vi "Read VISA address.vi"(8 "error in (no error)":errorcluster, 11 "PS Driver in":refnum<class "PS Driver.lvclass">) -> (0 "error out":errorcluster, 2 "VISA address":refnum<visa-resource-name>="GPIB0::22::INSTR", 3 "PS Driver out":refnum<class "PS Driver.lvclass">)   [LabVIEW 2021, in "PS Driver.lvlib" / "PS Driver.lvclass"]
uses:
  PS Driver.lvclass
  PS Driver.lvclass/PS Driver.ctl
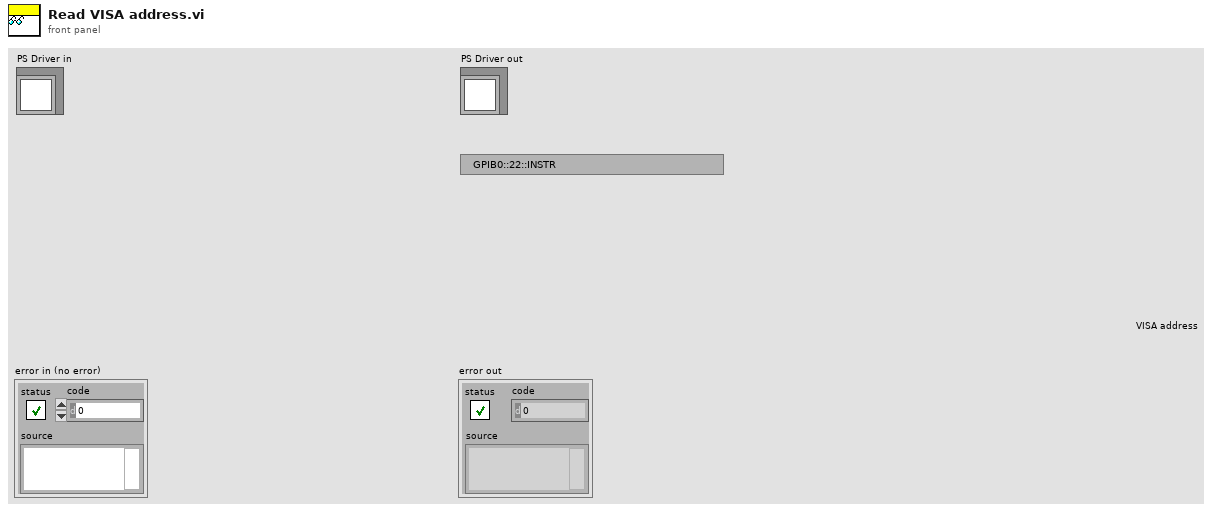
[diagram p1: front panel]
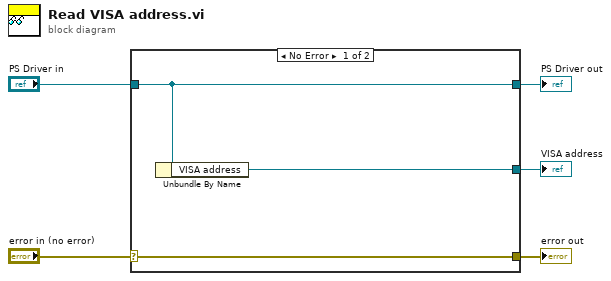
[diagram p0: block diagram]
diagram:
  n1 = case shown="No Error" "error in (no error)" {
    selector: "error in (no error)" -> [w8 w9]
    tunnel: [w8 w9] -> w4
    tunnel: [w7 w10] -> w2
    tunnel: "PS Driver in" -> [w7 w10]
    tunnel: [w6 _] -> w1
    frame No Error {
      n2 = Unbundle By Name(w7) -> ("VISA address"=w6:refnum<visa-resource-name>)
    }
    frame Error {
    }
  }
  "error out" <- w4
  "PS Driver out" <- w2
  "VISA address" <- w1
